vi "fpga.vi"() -> ()   [LabVIEW 2019]
doc: "Simple VI that sends analog input data back to host through a front panel indicator."
uses:
  <vilib>/rvi/Emulation/niFpgaGetClockAttributes.vi
  <vilib>/rvi/Emulation/niFpgaSctlEmulationGetInTimedLoop.vi
  <vilib>/rvi/Emulation/niFpgaEmulationReportErrorSimple.vi
  <vilib>/rvi/Emulation/niFpgaProcessEmulError.vi
  <vilib>/rvi/Emulation/niFpgaCriticalErrorInLSC.vi
  <vilib>/rvi/Emulation/niFpgaEmulationIsFPGAContextNoSignature.vi
  <vilib>/rvi/DataTransferAndStorage/Container/Common/niFpgaContainerGetUniqueNameForEmu.vi
  <vilib>/rvi/Memory/Memory_Emulation/niFpgaMemoryEmulationCacheClearOnFirstRun.vi
  <vilib>/rvi/Memory/Memory_Emulation/nirvimemoryEmulationManagerCache_MakeExclusive.vi
  <vilib>/rvi/Memory/Memory_Emulation/niFpgaMemoryEmulationValidateCache.vi
  <vilib>/rvi/Memory/Memory_Emulation/nirvimemoryEmulationManagerCache_InsertValue.vi
  <vilib>/Utility/error.llb/Clear Errors.vi
  <vilib>/rvi/Memory/Memory_Emulation/nirvimemoryEmulationManagerCache_ReleaseExclusive.vi
  <vilib>/rvi/Memory/Memory_Emulation/nirvimemoryEmulationManagerCache_GetValue.vi
  <vilib>/rvi/Memory/Memory_Emulation/nirvimemoryEmulationManagerCache_SetValue.vi
  sub/rti.global.vi
  <vilib>/rvi/eio/common/nirviEmuTemplateMethod_errors.vi
  <vilib>/rvi/DataTransferAndStorage/Container/XNode/niFpgaContainer.xnode
  <vilib>/rvi/DataTransferAndStorage/Register/Emulation/niFpgaRegisterEmulation.vi
  <vilib>/eio/EIONode/EIONode.xnode
panel:
  out "homed?":bool
  out "Chassis Temperature":i16
  out "config out":T1
  out "homing wait counter":u32
  in  "az pos req":fxp<+/-,32,2>
  out "homing?":bool
  in  "config":T1={"io.cloud-enable"=FALSE, "io.encoder-negate"=FALSE, "io.encoder-ref"=79895940197, "io.encoder-step"=4018143232, "io.home-pos"=0.0, "sm.az-timeout (ms)"=120000, "sm.encoder-no-error"=1025, "sm.main-pos-hs-thres"=0.013888888992369175, "sm.main-pos-tol"=0.00138888880610466, "sm.cloud-timeout (ms)"=100000, "sm.rev-dly (ms)"=4000, "io.encoder-center"=68719476735, "sm-main-center-hs-thres"=55807545, "sm-main-center-tol"=5580754}
  out "cmd":i8
  out "cmd request":i8
  out "rev dly counter":u32
  out "home sensor":bool
  out "env sensor":bool
  out "az to counter":u32
  out "cloud to counter":u32
  out "cloud?":bool
  out "buttons":T2
  out "enc status":u16
  out "sub mode":u8
  out "mode":u8
  out "az pos":fxp<+/-,32,2>
  out "az enc counts":u64
  out "errors":T3
  out "error?":bool
  in  "emergency stop":bool
  out "az last rotation":enum16{"none", "forward", "reverse"}(ring)
  in  "mode request":enum16{"stop", "home", "position", "center"}(ring)
  in  "reset":bool
  out "rs":bool
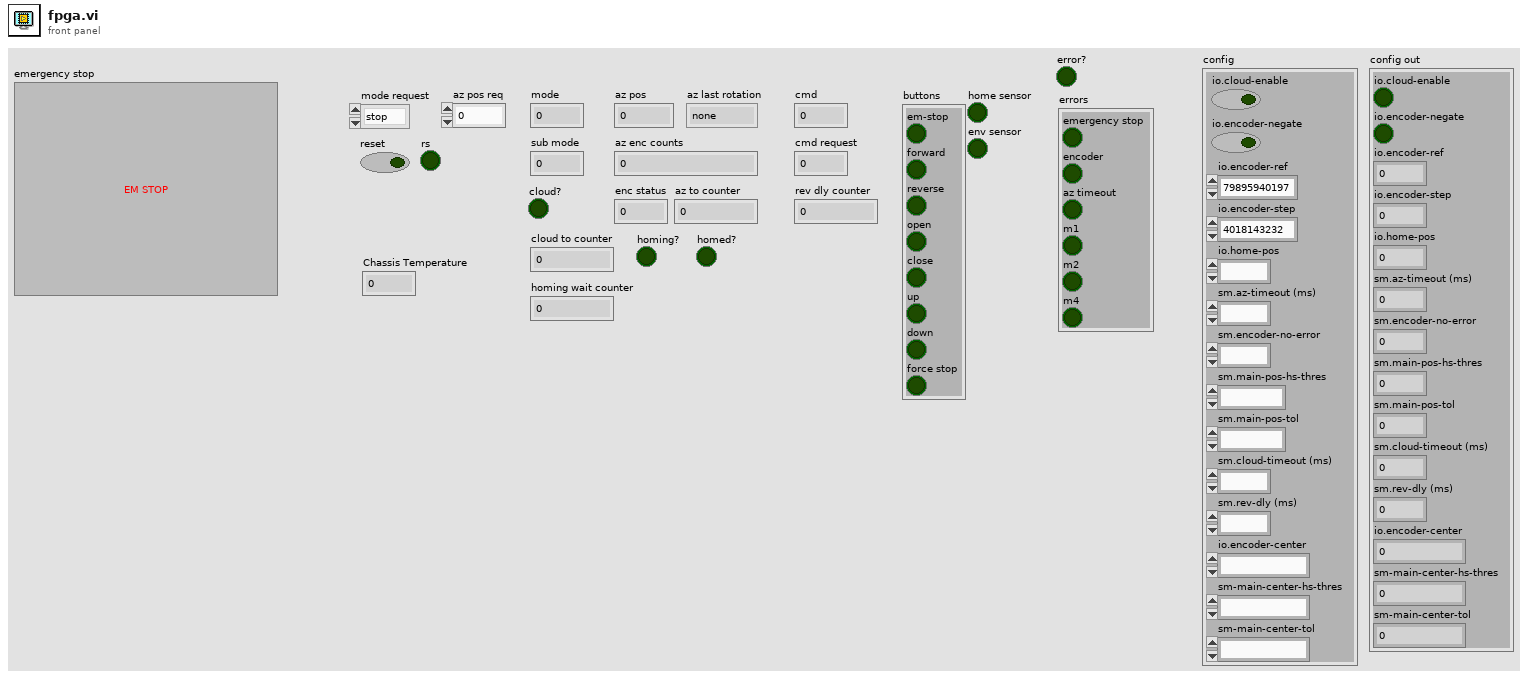
[diagram p1: front panel]
types:
  T1 = cluster{"io.cloud-enable":bool, "io.encoder-negate":bool, "io.encoder-ref":u64, "io.encoder-step":u64, "io.home-pos":fxp<+/-,32,2>, "sm.az-timeout (ms)":u32, "sm.encoder-no-error":u16, "sm.main-pos-hs-thres":fxp<+/-,32,2>, "sm.main-pos-tol":fxp<+/-,32,2>, "sm.cloud-timeout (ms)":u32, "sm.rev-dly (ms)":u32, "io.encoder-center":u64, "sm-main-center-hs-thres":u64, "sm-main-center-tol":u64}
  T2 = cluster{"em-stop":bool, "forward":bool, "reverse":bool, "open":bool, "close":bool, "up":bool, "down":bool, "force stop":bool}
  T3 = cluster{"emergency stop":bool, "encoder":bool, "az timeout":bool, "m1":bool, "m2":bool, "m4":bool}
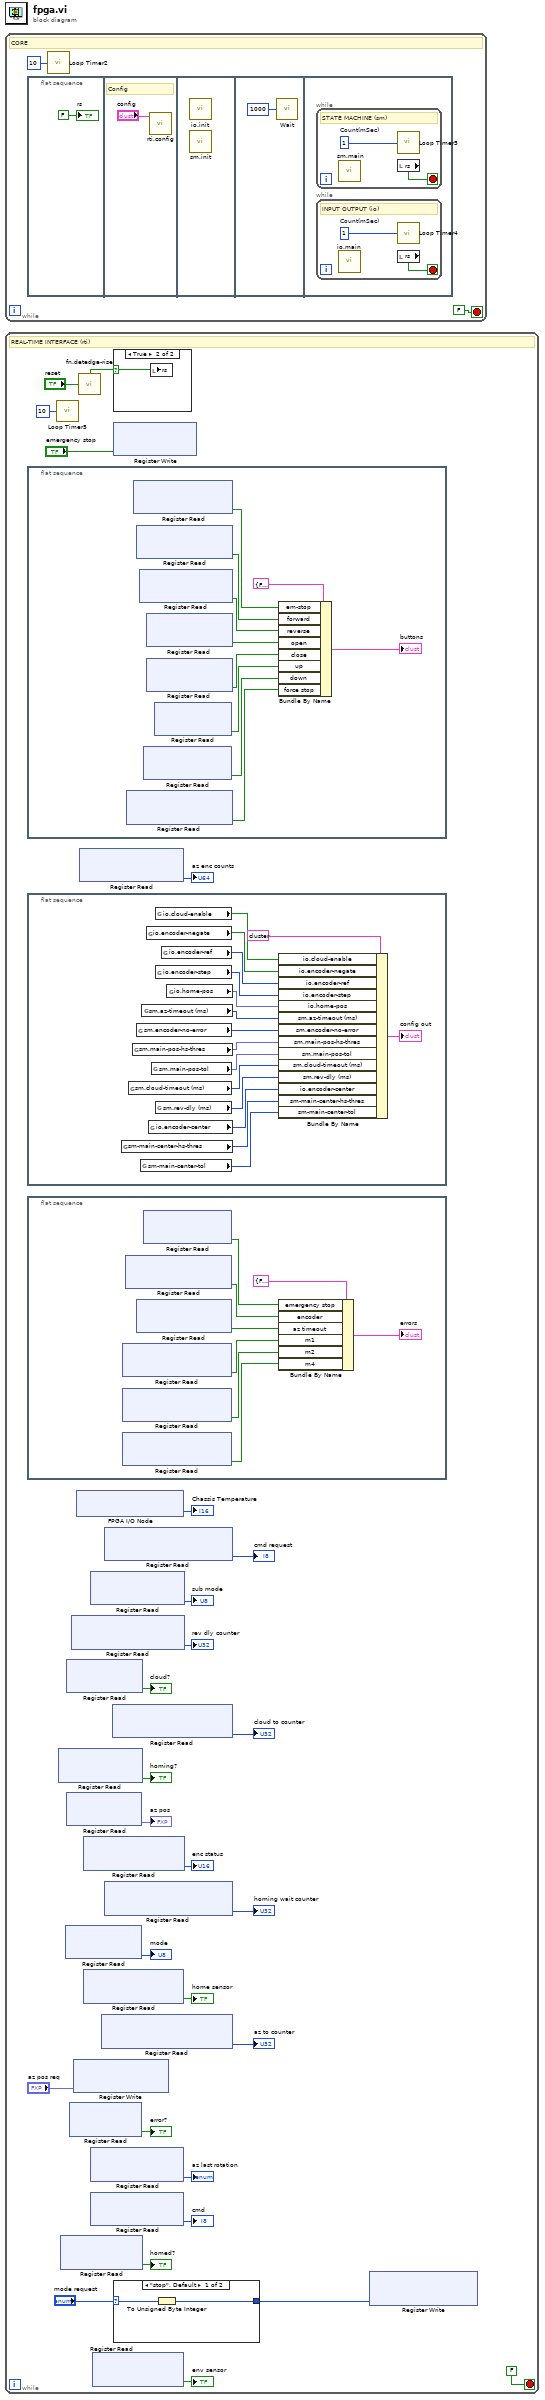
[diagram p0: block diagram]
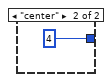
[diagram p2: hidden frame]
diagram:
  n1 = while {
    stop <- FALSE stop-if-true
    # "CORE"
    n2 = flat-sequence {
      frame #0 {
        "rs" <- FALSE ("rs")
      }
      frame #1 {
        # "Config"
        n3 = call "rti.config"("config"="config") -> ()  [unwired: 11 in]
      }
      frame #2 {
        n4 = call "io.init.vi"() -> ()  [unwired: 12 in]
        n5 = call "sm.init.vi"() -> ()  [unwired: 12 in]
      }
      frame #3 {
        n6 = call "Wait"("Count(mSec)"=u16 1000 ("Count(uSec)")) -> ()  [unwired: 1 out]
      }
      frame #4 {
        n7 = while {
          stop <- w9 stop-if-true
          w8 = u16 1  # Count(mSec)
          # "STATE MACHINE (sm)"
          n8 = call "sm.main.vi"() -> ()  [unwired: 12 in]
          n9 = call "Loop Timer3"("Count(mSec)"=w8) -> ()  [unwired: 1 out]
          n10 = local read "rs"() -> (w9:bool)
        }
        n11 = while {
          stop <- w7 stop-if-true
          w6 = u16 1  # Count(mSec)
          # "INPUT OUTPUT (io)"
          n12 = call "io.main.vi"() -> ()  [unwired: 12 in]
          n13 = call "Loop Timer4"("Count(mSec)"=w6) -> ()  [unwired: 1 out]
          n14 = local read "rs"() -> (w7:bool)
        }
      }
    }
    n15 = call "Loop Timer2"("Count(mSec)"=u16 10 ("Count(uSec)")) -> ()  [unwired: 1 out]
  }
  n16 = while {
    stop <- FALSE stop-if-true
    # "REAL-TIME INTERFACE (rti)"
    n17 = flat-sequence {
      frame #0 {
        n18 = xnode ("Register Read")() -> ("Data"=w40:bool)  [unwired: 1 in, 1 out]
        n19 = xnode ("Register Read")() -> ("Data"=w42:bool)  [unwired: 1 in, 1 out]
        n20 = xnode ("Register Read")() -> ("Data"=w43:bool)  [unwired: 1 in, 1 out]
        n21 = xnode ("Register Read")() -> ("Data"=w44:bool)  [unwired: 1 in, 1 out]
        n22 = xnode ("Register Read")() -> ("Data"=w48:bool)  [unwired: 1 in, 1 out]
        n23 = xnode ("Register Read")() -> ("Data"=w45:bool)  [unwired: 1 in, 1 out]
        n24 = xnode ("Register Read")() -> ("Data"=w46:bool)  [unwired: 1 in, 1 out]
        n25 = xnode ("Register Read")() -> ("Data"=w47:bool)  [unwired: 1 in, 1 out]
        n26 = Bundle By Name(cluster=T2 {"em-stop"=FALSE, "forward"=FALSE, "reverse"=FALSE, "open"=FALSE, "close"=FALSE, "up"=FALSE, "down"=FALSE, "force stop"=FALSE}, "em-stop"=w42, "forward"=w43, "reverse"=w44, "open"=w45, "close"=w46, "up"=w47, "down"=w48, "force stop"=w40) -> (→"buttons":T2)
      }
    }
    n27 = flat-sequence {
      frame #0 {
        n28 = global read "rti.global.vi" "sm-main-center-hs-thres"() -> (w59:u64)
        n29 = global read "rti.global.vi" "sm.cloud-timeout (ms)"() -> (w62:u32)
        n30 = global read "rti.global.vi" "sm.main-pos-hs-thres"() -> (w64:fxp<+/-,32,2>)
        n31 = global read "rti.global.vi" "sm.encoder-no-error"() -> (w65:u16)
        n32 = global read "rti.global.vi" "sm-main-center-tol"() -> (w58:u64)
        n33 = global read "rti.global.vi" "sm.az-timeout (ms)"() -> (w66:u32)
        n34 = global read "rti.global.vi" "io.encoder-negate"() -> (w70:bool)
        n35 = global read "rti.global.vi" "io.encoder-center"() -> (w60:u64)
        n36 = global read "rti.global.vi" "sm.main-pos-tol"() -> (w63:fxp<+/-,32,2>)
        n37 = global read "rti.global.vi" "io.cloud-enable"() -> (w71:bool)
        n38 = global read "rti.global.vi" "io.encoder-step"() -> (w68:u64)
        n39 = global read "rti.global.vi" "sm.rev-dly (ms)"() -> (w61:u32)
        n40 = global read "rti.global.vi" "io.encoder-ref"() -> (w69:u64)
        n41 = global read "rti.global.vi" "io.home-pos"() -> (w67:fxp<+/-,32,2>)
        n42 = Bundle By Name(cluster=T1 {"io.cloud-enable"=FALSE, "io.encoder-negate"=FALSE, "io.encoder-ref"=79895940197, "io.encoder-step"=4018143232, "io.home-pos"=0.0, "sm.az-timeout (ms)"=120000, "sm.encoder-no-error"=1025, "sm.main-pos-hs-thres"=0.013888888992369175, "sm.main-pos-tol"=0.00138888880610466, "sm.cloud-timeout (ms)"=100000, "sm.rev-dly (ms)"=4000, "io.encoder-center"=68719476735, "sm-main-center-hs-thres"=55807545, "sm-main-center-tol"=5580754} ("config"), "io.cloud-enable"=w71, "io.encoder-negate"=w70, "io.encoder-ref"=w69, "io.encoder-step"=w68, "io.home-pos"=w67, "sm.az-timeout (ms)"=w66, "sm.encoder-no-error"=w65, "sm.main-pos-hs-thres"=w64, "sm.main-pos-tol"=w63, "sm.cloud-timeout (ms)"=w62, "sm.rev-dly (ms)"=w61, "io.encoder-center"=w60, "sm-main-center-hs-thres"=w59, "sm-main-center-tol"=w58) -> (→"config out":T1)
      }
    }
    n43 = flat-sequence {
      frame #0 {
        n44 = xnode ("Register Read")() -> ("Data"=w54:bool)  [unwired: 1 in, 1 out]
        n45 = xnode ("Register Read")() -> ("Data"=w55:bool)  [unwired: 1 in, 1 out]
        n46 = xnode ("Register Read")() -> ("Data"=w56:bool)  [unwired: 1 in, 1 out]
        n47 = xnode ("Register Read")() -> ("Data"=w52:bool)  [unwired: 1 in, 1 out]
        n48 = xnode ("Register Read")() -> ("Data"=w53:bool)  [unwired: 1 in, 1 out]
        n49 = xnode ("Register Read")() -> ("Data"=w51:bool)  [unwired: 1 in, 1 out]
        n50 = Bundle By Name(cluster=T3 {"emergency stop"=FALSE, "encoder"=FALSE, "az timeout"=FALSE, "m1"=FALSE, "m2"=FALSE, "m4"=FALSE}, "emergency stop"=w51, "encoder"=w52, "az timeout"=w53, "m1"=w54, "m2"=w55, "m4"=w56) -> (→"errors":T3)
      }
    }
    n51 = call "Loop Timer5"("Count(mSec)"=u8 10 ("Count(uSec)")) -> ()  [unwired: 1 out]
    n52 = xnode ("Register Read")() -> ("Data"=→"homing?":bool)  [unwired: 1 in, 1 out]
    n53 = xnode ("Register Read")() -> ("Data"=→"homed?":bool)  [unwired: 1 in, 1 out]
    n54 = xnode ("Register Read")() -> ("Data"=→"mode":u8)  [unwired: 1 in, 1 out]
    n55 = xnode ("Register Read")() -> ("Data"=→"cloud?":bool)  [unwired: 1 in, 1 out]
    n56 = xnode ("Register Read")() -> ("Data"=→"az pos":fxp<+/-,32,2>)  [unwired: 1 in, 1 out]
    n57 = xnode ("Register Read")() -> ("Data"=→"error?":bool)  [unwired: 1 in, 1 out]
    n58 = xnode ("Register Read")() -> ("Data"=→"rev dly counter":u32)  [unwired: 1 in, 1 out]
    n59 = xnode ("Register Write")("Data"="az pos req") -> ()  [unwired: 1 in, 1 out]
    n60 = xnode "FPGA I/O Node"() -> ("Chassis Temperature"=→"Chassis Temperature":i16)  [unwired: 1 in, 1 out]
    n61 = call "fn.detedge-rise.vi"("Signal in"="reset") -> ("Edge?"=w34:bool)  [unwired: 2 in, 1 out]
    n62 = xnode ("Register Read")() -> ("Data"=→"az enc counts":u64)  [unwired: 1 in, 1 out]
    n63 = xnode ("Register Read")() -> ("Data"=→"enc status":u16)  [unwired: 1 in, 1 out]
    n64 = xnode ("Register Read")() -> ("Data"=→"home sensor":bool)  [unwired: 1 in, 1 out]
    n65 = xnode ("Register Read")() -> ("Data"=→"sub mode":u8)  [unwired: 1 in, 1 out]
    n66 = xnode ("Register Read")() -> ("Data"=→"az last rotation":u8)  [unwired: 1 in, 1 out]
    n67 = xnode ("Register Read")() -> ("Data"=→"cmd":i8)  [unwired: 1 in, 1 out]
    n68 = xnode ("Register Read")() -> ("Data"=→"env sensor":bool)  [unwired: 1 in, 1 out]
    n69 = xnode ("Register Read")() -> ("Data"=→"az to counter":u32)  [unwired: 1 in, 1 out]
    n70 = xnode ("Register Read")() -> ("Data"=→"cmd request":i8)  [unwired: 1 in, 1 out]
    n71 = xnode ("Register Read")() -> ("Data"=→"homing wait counter":u32)  [unwired: 1 in, 1 out]
    n72 = xnode ("Register Read")() -> ("Data"=→"cloud to counter":u32)  [unwired: 1 in, 1 out]
    n73 = case shown="True" w34 {
      selector: w34 -> [_ w74]
      frame False {
      }
      frame True {
        n74 = local write "rs"(w74) -> ()
      }
    }
    n75 = xnode ("Register Write")("Data"="emergency stop") -> ()  [unwired: 1 in, 1 out]
    n76 = case shown="\"stop\", Default" "mode request" {
      selector: "mode request" -> [w37 _]
      tunnel: [w38 u8 4] -> w12
      frame "stop", Default {
        n77 = To Unsigned Byte Integer(number=w37) -> (unsigned 8bit integer=w38:u8)
      }
      frame "center" {
      }
    }
    n78 = xnode ("Register Write")("Data"=w12) -> ()  [unwired: 1 in, 1 out]
  }
